vi "Match_Score.vi"(11 "before match in":string) -> (3 "number":dbl)   [LabVIEW 2019]
uses:
  <vilib>/regexp/Match Regular Expression.xnode
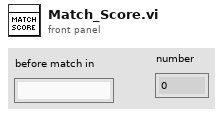
[diagram p1: front panel]
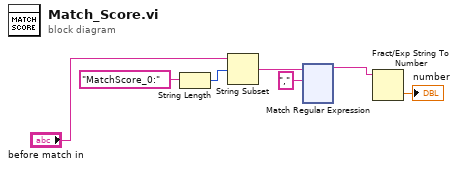
[diagram p0: block diagram]
diagram:
  n1 = String Length(string="MatchScore_0:") -> (length=w6:i32)
  n2 = String Subset(string="before match in", offset (0)=w6) -> (substring=w4:string)  [unwired: 1 in]
  n3 = xnode "Match Regular Expression"("input string"=w4, "regular expression"=",") -> ("before match"=w2:string)  [unwired: 4 in, 4 out]
  n4 = Fract/Exp String To Number(string=w2) -> (number=→"number":dbl)  [unwired: 3 in, 1 out]
